vi "clearpath_parse_platform_info.vi"(0 "ClearpathComm":T1) -> (1 "Data Valid":bool=TRUE, 2 "Revision":i32, 3 "Serial":i32, 4 "Model":string)   [LabVIEW 2010, in "clearpath_interface.lvlib"]
doc: "Parses general platform information as returned by platform. (Message type 0x8001)"
uses:
  clearpath_interface.lvlib
  cwrap_cRIO.dll
panel:
  # "Platform Info"
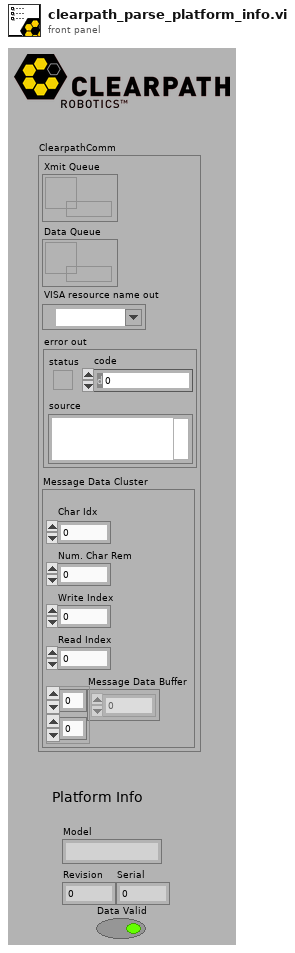
[diagram p1: front panel]
types:
  T1 = cluster{"Xmit Queue":refnum<queue>, "Data Queue":refnum<queue>, "VISA resource name out":refnum<visa-resource-name>, "error out":errorcluster, "Message Data Cluster":cluster{"\nChar Idx":u8, "Num. Char Rem":u8, "Write Index":u8, "Read Index":u8, "Message Data Buffer":u8[][]}}
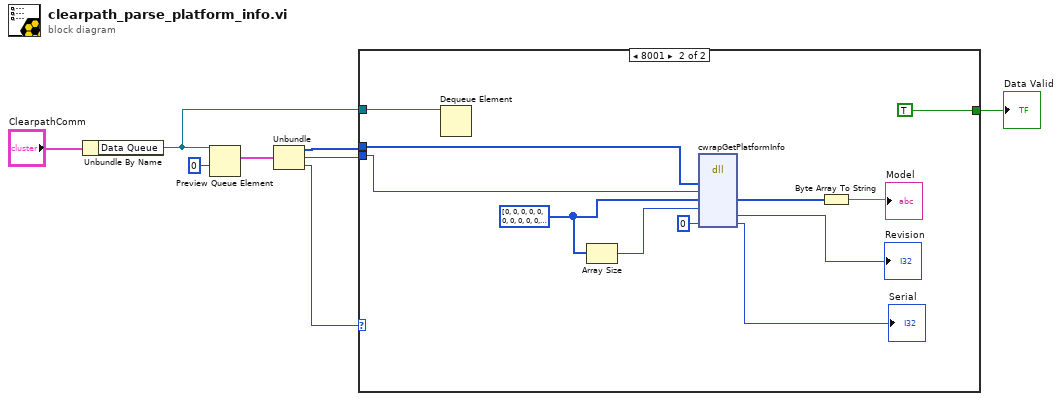
[diagram p0: block diagram]
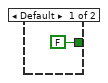
[diagram p2: hidden frame]
diagram:
  n1 = Unbundle By Name("ClearpathComm") -> ("Data Queue"=w2:refnum<queue>)
  n2 = Preview Queue Element(queue=w2, timeout in ms (-1)=0) -> (element=w1:cluster{u8[], "Length":i32, "Type":i32})  [unwired: 1 in, 3 out]
  n3 = Unbundle(w1) -> (w4:u8[], "Length"=w5:i32, "Type"=w6:i32)
  n4 = case shown="8001" w6 {
    tunnel: w5 -> [_ w12]
    tunnel: w4 -> [_ w13]
    tunnel: [FALSE TRUE] -> w3
    tunnel: w2 -> [_ w10]
    frame Default {
    }
    frame 32769 {
      w20 = i32[] [0, 0, 0, 0, 0, 0, 0, 0, 0, 0, 0, 0] ("Array")
      n5 = Dequeue Element(queue=w10) -> ()  [unwired: 2 in, 4 out]
      n6 = Array Size(array=w20) -> (size(s)=w19:i32)
      n7 = dll-call lib="cwrap_cRIO.*" fn="cwrapGetPlatformInfo"("packet"=w13, "len"=w12, "model"=w20, "name_len"=w19, "serial"=0) -> ("model"=w18:i8[], "revision"=→"Revision":i8, "serial"=→"Serial":i32)  [unwired: 8 in, 2 out]
      n8 = Byte Array To String(unsigned byte array=w18) -> (string=→"Model":string)
    }
  }
  "Data Valid" <- w3
